vi "get dependency list.vi"(8 "error in":errorcluster, 11 "CVT Engine Editor in":refnum<class "CVT Engine Editor.lvclass">) -> (0 "error out":errorcluster, 2 "files":T1[](array[typedef]), 3 "CVT Engine Editor out":refnum<class "CVT Engine Editor.lvclass">)   [LabVIEW 2013, in "CVT Engine Editor.lvclass"]
uses:
  CVT Engine Editor.lvclass
  <vilib>/NI/Tag Bus Data Framework/Configuration Editor/Classes/TBM Configuration Node/deployment configuration.ctl
  <vilib>/NI/Tag Bus Data Framework/Configuration Editor/Classes/Engine Parent/Engine Parent Editor Node.lvclass
  <vilib>/NI/Tag Bus Data Framework/Configuration Editor/Classes/TBM Configuration Node/TBM Configuration Node.lvclass
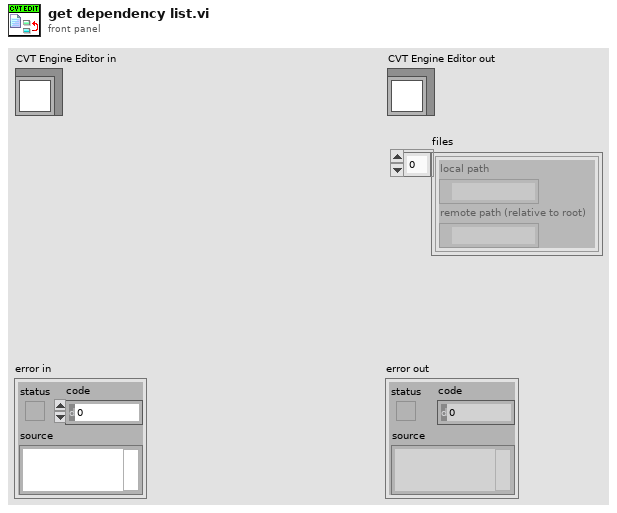
[diagram p1: front panel]
types:
  T1 = typedef "PL Framework Configuration Tool.lvlib/TBM Configuration Node.lvclass/deployment configuration.ctl" = cluster{"local path":path, "remote path (relative to root)":path}
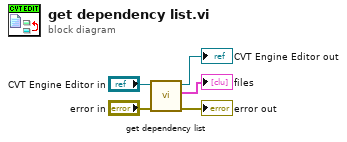
[diagram p0: block diagram]
diagram:
  n1 = call-parent "get dependency list.vi"("error in"="error in", "TBM Configuration Node in"="CVT Engine Editor in") -> ("error out"=→"error out":errorcluster, "files"=→"files":T1[], "TBM Configuration Node out"=→"CVT Engine Editor out":refnum<class "CVT Engine Editor.lvclass">)  [unwired: 7 in]
